vi "2 step.vi"(0 "УЗ2":dbl format="%#_13g", 5 "УЗ3":dbl format="%#_13g", 7 "ДМ1":dbl format="%#_13g", 9 "Error input":bool=TRUE) -> (4 "Насос 2":bool=TRUE, 6 "ДН2":bool=TRUE, 8 "Донный клапан":bool=TRUE, 10 "объем подачи ДН2":dbl format="%#_13g", 15 "Error output":bool=TRUE)   [LabVIEW 2019]
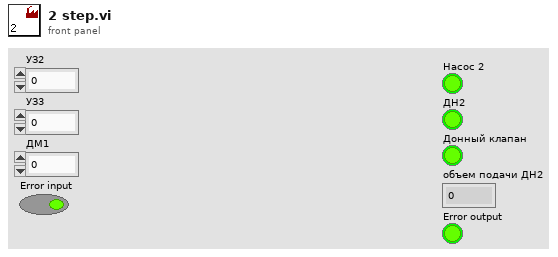
[diagram p1: front panel]
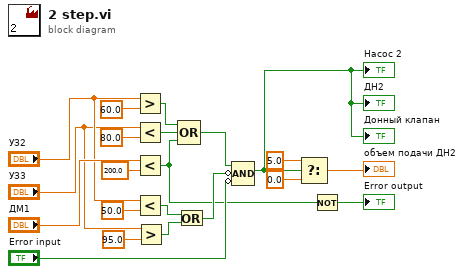
[diagram p0: block diagram]
diagram:
  n1 = Greater?(x="УЗ2", y=60.0) -> (0:w18:bool)
  n2 = Less?(x="УЗ3", y=80.0) -> (x < y?=w17:bool)
  n3 = Less?(x="ДМ1", y=200.0) -> (x < y?=w1:bool)
  n4 = Less?(x="УЗ2", y=50.0) -> (x < y?=w9:bool)
  n5 = Greater?(x="УЗ3", y=95.0) -> (0:w8:bool)
  n6 = Or(x=w9, y=w8) -> (x .or. y?=w7:bool)
  n7 = Compound Arithmetic op=OR(w18, w17, w1) -> (w6:bool)
  n8 = Compound Arithmetic op=AND(w6, invert w7, invert "Error input") -> (w5:bool)
  "Насос 2" <- w5
  "ДН2" <- w5
  "Донный клапан" <- w5
  n9 = Select(t=5.0, s=w5, f=0.0) -> (s? t:f=→"объем подачи ДН2":dbl)
  n10 = Not(x=w1) -> (.not. x?=→"Error output":bool)
